vi "Wheel_detector_status.vi"(8 "WD_offset":dbl=0.003, 9 "I2":sgl[](array[numeric])=array[5000 elements], 10 "I1":sgl[](array[numeric])=array[5000 elements], 11 "Direccion 0?":bool) -> (1 "WD_status":string, 2 "I2":bool, 3 "I1":bool)   [LabVIEW 2015]
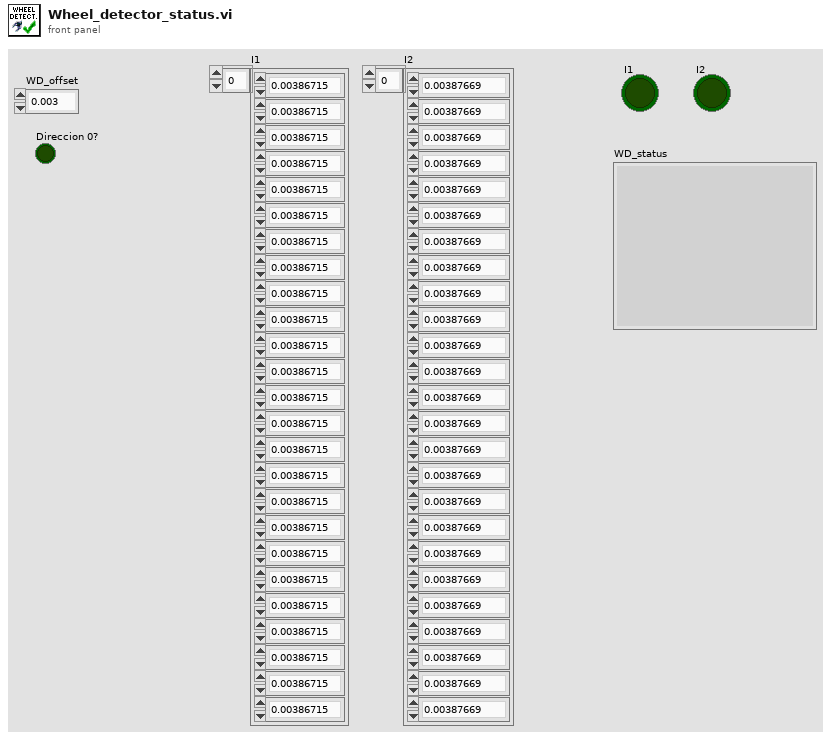
[diagram p1: front panel]
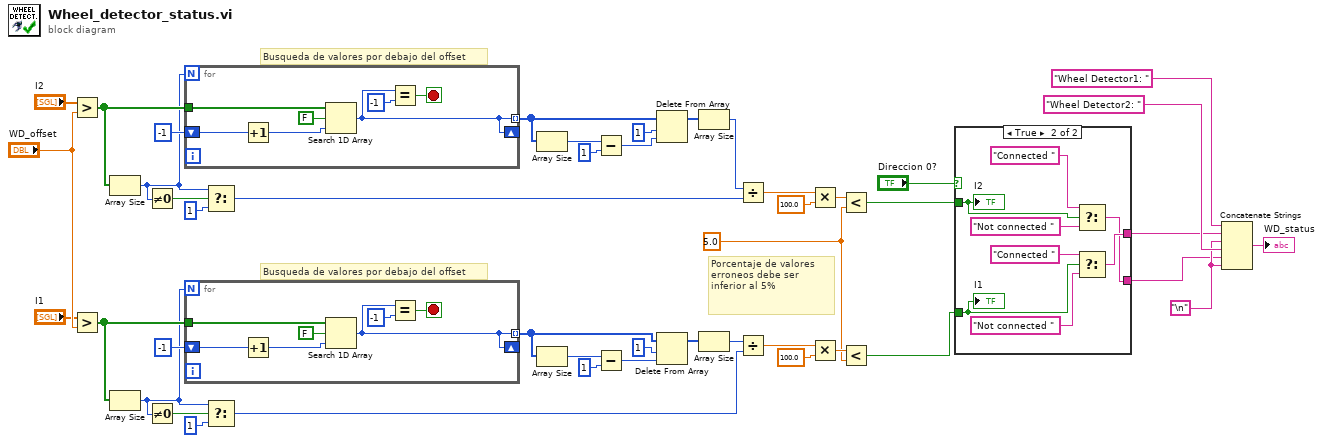
[diagram p0: block diagram]
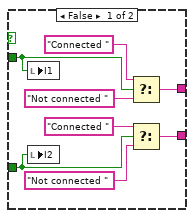
[diagram p2: hidden frame]
diagram:
  w7 = "\n"
  w3 = 5.0 ("y")
  # "Busqueda de valores por debajo del offset"
  # "Porcentaje de valores erroneos debe ser inferior al 5%"
  # "Busqueda de valores por debajo del offset"
  n1 = Greater?(x="I2", y="WD_offset") -> (0:w33:bool[])
  n2 = Greater?(x="I1", y="WD_offset") -> (0:w45:bool[])
  n3 = Array Size(array=w33) -> (size(s)=w25:i32)
  n4 = Array Size(array=w45) -> (size(s)=w37:i32)
  n5 = Not Equal To 0?(x=w25) -> (x != 0?=w30:bool)
  n6 = Not Equal To 0?(x=w37) -> (x != 0?=w42:bool)
  n7 = for {
    N: w25 -> [_]
    tunnel: w33 -> [w52]
    tunnel: [w49] -> w12 mode=indexing
    shift-right: [w49] -> _
    shift-left: -1 ("index of element") -> [w47]
    stop <- w50 stop-if-true
    n8 = Increment(x=w47) -> (x+1=w46:i32)
    n9 = Search 1D Array(1D array=w52, element=FALSE, start index (0)=w46) -> (index of element=w49:i32)
    n10 = Equal?(x=w49, y=-1) -> (x = y?=w50:bool)
  }
  n11 = for {
    N: w37 -> [_]
    tunnel: w45 -> [w59]
    tunnel: [w56] -> w17 mode=indexing
    shift-right: [w56] -> _
    shift-left: -1 ("index of element") -> [w54]
    stop <- w57 stop-if-true
    n12 = Increment(x=w54) -> (x+1=w53:i32)
    n13 = Search 1D Array(1D array=w59, element=FALSE, start index (0)=w53) -> (index of element=w56:i32)
    n14 = Equal?(x=w56, y=-1) -> (x = y?=w57:bool)
  }
  n15 = Select(t=w25, s=w30, f=1) -> (s? t:f=w31:i32)
  n16 = Select(t=w37, s=w42, f=1) -> (s? t:f=w43:i32)
  n17 = Array Size(array=w12) -> (size(s)=w16:i32)
  n18 = Array Size(array=w17) -> (size(s)=w22:i32)
  n19 = Subtract(x=w16, y=1 ("length")) -> (x-y=w14:i32)
  n20 = Subtract(x=w22, y=1 ("length")) -> (x-y=w20:i32)
  n21 = Delete From Array(array=w12, length=1, index=w14) -> (array with subset deleted=w11:i32[])  [unwired: 1 out]
  n22 = Delete From Array(array=w17, length=1, index=w20) -> (array with subset deleted=w18:i32[])  [unwired: 1 out]
  n23 = Array Size(array=w11) -> (size(s)=w26:i32)
  n24 = Array Size(array=w18) -> (size(s)=w38:i32)
  n25 = Divide(x=w26, y=w31) -> (x/y=w28:dbl)
  n26 = Divide(x=w38, y=w43) -> (x/y=w40:dbl)
  n27 = Multiply(x=w28, y=100.0) -> (x*y=w24:dbl)
  n28 = Multiply(x=w40, y=100.0) -> (x*y=w35:dbl)
  n29 = Less?(x=w24, y=w3) -> (x < y?=w10:bool)
  n30 = Less?(x=w35, y=w3) -> (x < y?=w34:bool)
  n31 = case shown="True" "Direccion 0?" {
    tunnel: w34 -> [w63 w73]
    tunnel: w10 -> [w62 w70]
    tunnel: [w61 w69] -> w6
    tunnel: [w60 w68] -> w5
    frame False {
      n32 = local write "I1"(w62) -> ()
      n33 = local write "I2"(w63) -> ()
      n34 = Select(t="Connected " ("string"), s=w62, f="Not connected " ("string")) -> (s? t:f=w61:string)
      n35 = Select(t="Connected " ("string"), s=w63, f="Not connected " ("string")) -> (s? t:f=w60:string)
    }
    frame True {
      n36 = Select(t="Connected " ("string"), s=w70, f="Not connected " ("string")) -> (s? t:f=w68:string)
      n37 = Select(t="Connected " ("string"), s=w73, f="Not connected " ("string")) -> (s? t:f=w69:string)
      "I1" <- w73
      "I2" <- w70
    }
  }
  n38 = Concatenate Strings("Wheel Detector1: " ("string"), w6, w7, "Wheel Detector2: " ("string"), w5, w7) -> (→"WD_status":string)
